vi "UserVars-Randomize Values.vi"(7 "UserVars In":T1[](array[typedef]), 11 "error in (no error)":errorcluster) -> (8 "UserVars Out":T1[](array[typedef]), 15 "error out":errorcluster)   [LabVIEW 2020]
uses:
  User Variable.ctl
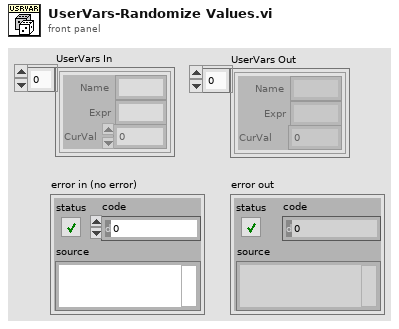
[diagram p1: front panel]
types:
  T1 = typedef "User Variable.ctl" = cluster{"Name":string, "Expr":string, "CurVal":dbl}
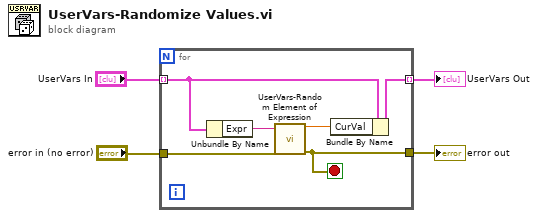
[diagram p0: block diagram]
diagram:
  n1 = for {
    tunnel: "UserVars In" -> [w10] mode=indexing
    tunnel: [w7] -> w3 mode=indexing
    tunnel: [w8] -> w2
    tunnel: "error in (no error)" -> [w5]
    stop <- w8 stop-if-true
    n2 = Unbundle By Name(w10) -> ("Expr"=w9:string)
    n3 = call "UserVars-Random Element of Expression.vi"("Expr"=w9, "error in (no error)"=w5) -> ("Random Element"=w6:dbl, "error out"=w8:errorcluster)  [unwired: 11 in, 1 out]
    n4 = Bundle By Name(cluster=w10, "CurVal"=w6) -> (w7:T1)
  }
  "UserVars Out" <- w3
  "error out" <- w2
